vi "sever-client.vi"() -> ()   [LabVIEW 2020]
uses:
  <vilib>/Utility/sysdir.llb/System Directory Type.ctl
panel:
  in  "s 6":bool=TRUE
  in  "s 5":bool
  in  "s 4":bool=TRUE
  in  "批量发送菜单":bool
  out "接收数据":string
  in  "发送数据":string
  out "远程端口":u16
  out "远程地址":string
  in  "批量发送":string[][](table)=[["Date", "Delay(ms)"], ["", ""], ["", ""], ["", ""], ["", ""], ["", ""]]
  in  "定时间隔毫秒":dbl
  in  "定时发送":bool
  out "当前发送":string
  out "数值":dbl
  out "times":dbl
  in  "s 3":bool
  out "添加的路径":path
  out "每小时读码次数":dbl
  in  "s 2":bool
  out "时间统计":string
  in  "s":bool
  out "total times":dbl
  out "standard output":string caption="PING标准输出"
  in  "停止":bool
  in  "开启检测模式":bool
  out "误码次数":dbl
  in  "标准码词":string="\r"
  in  "十六进制显示":bool=TRUE
  in  "自动换行":bool=TRUE
  in  "时间显示":bool=TRUE
  in  "接收超时毫秒":i32=200
  in  "清空接收数据区":bool
  in  "读取的字节":i32=300
  in  "十六进制发送":bool=TRUE
  in  "清空发送数据区":bool
  in  "发送超时毫秒":i32=200
  in  "发送":bool
  in  "数据保存":bool
  in  "路径":path
  in  "服务器IP地址":string="192.168.1.103"
  in  "sever-client":u16(ring) items=["TCP-Sever", "TCP-client"]
  in  "服务器端口号":u16=34567
  in  "开始":bool
  out "错误输出":errorcluster caption="TCP错误输出"
  # "V1.0.1"
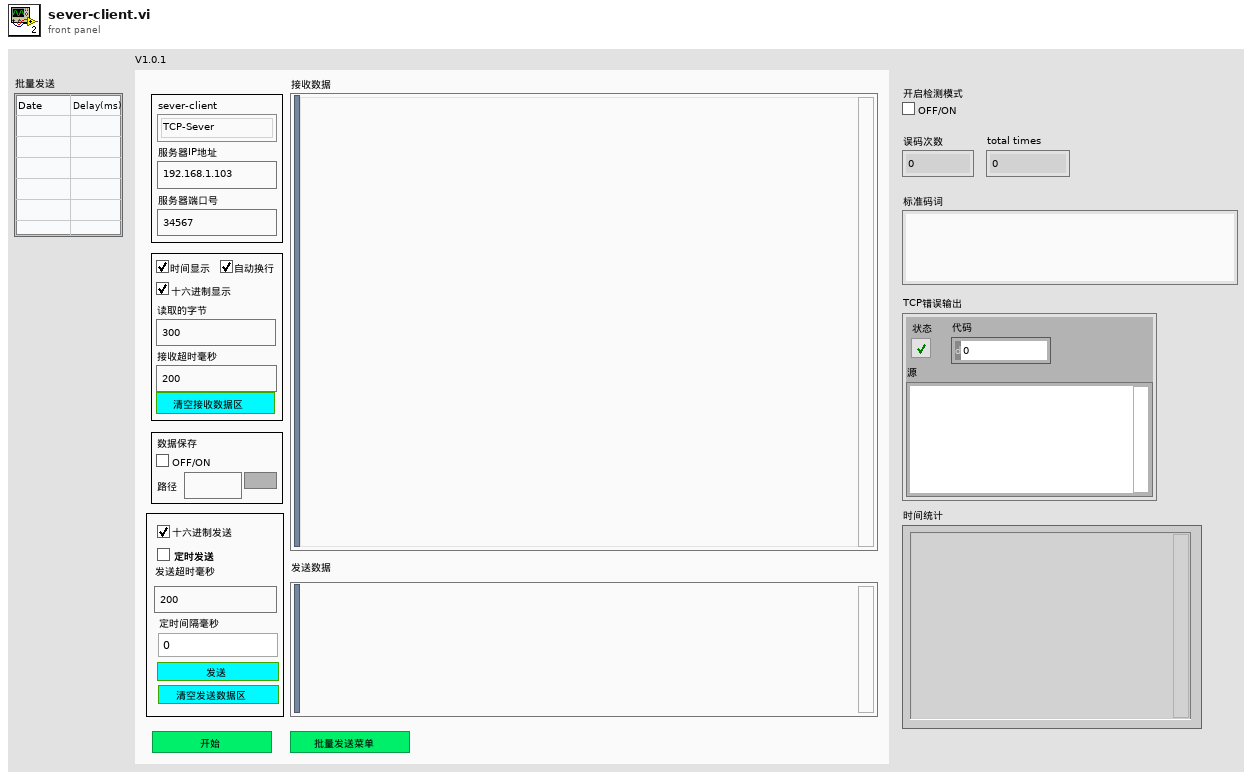
[diagram p1: front panel]
types:
  T1 = typedef "System Directory Type.ctl" = i32
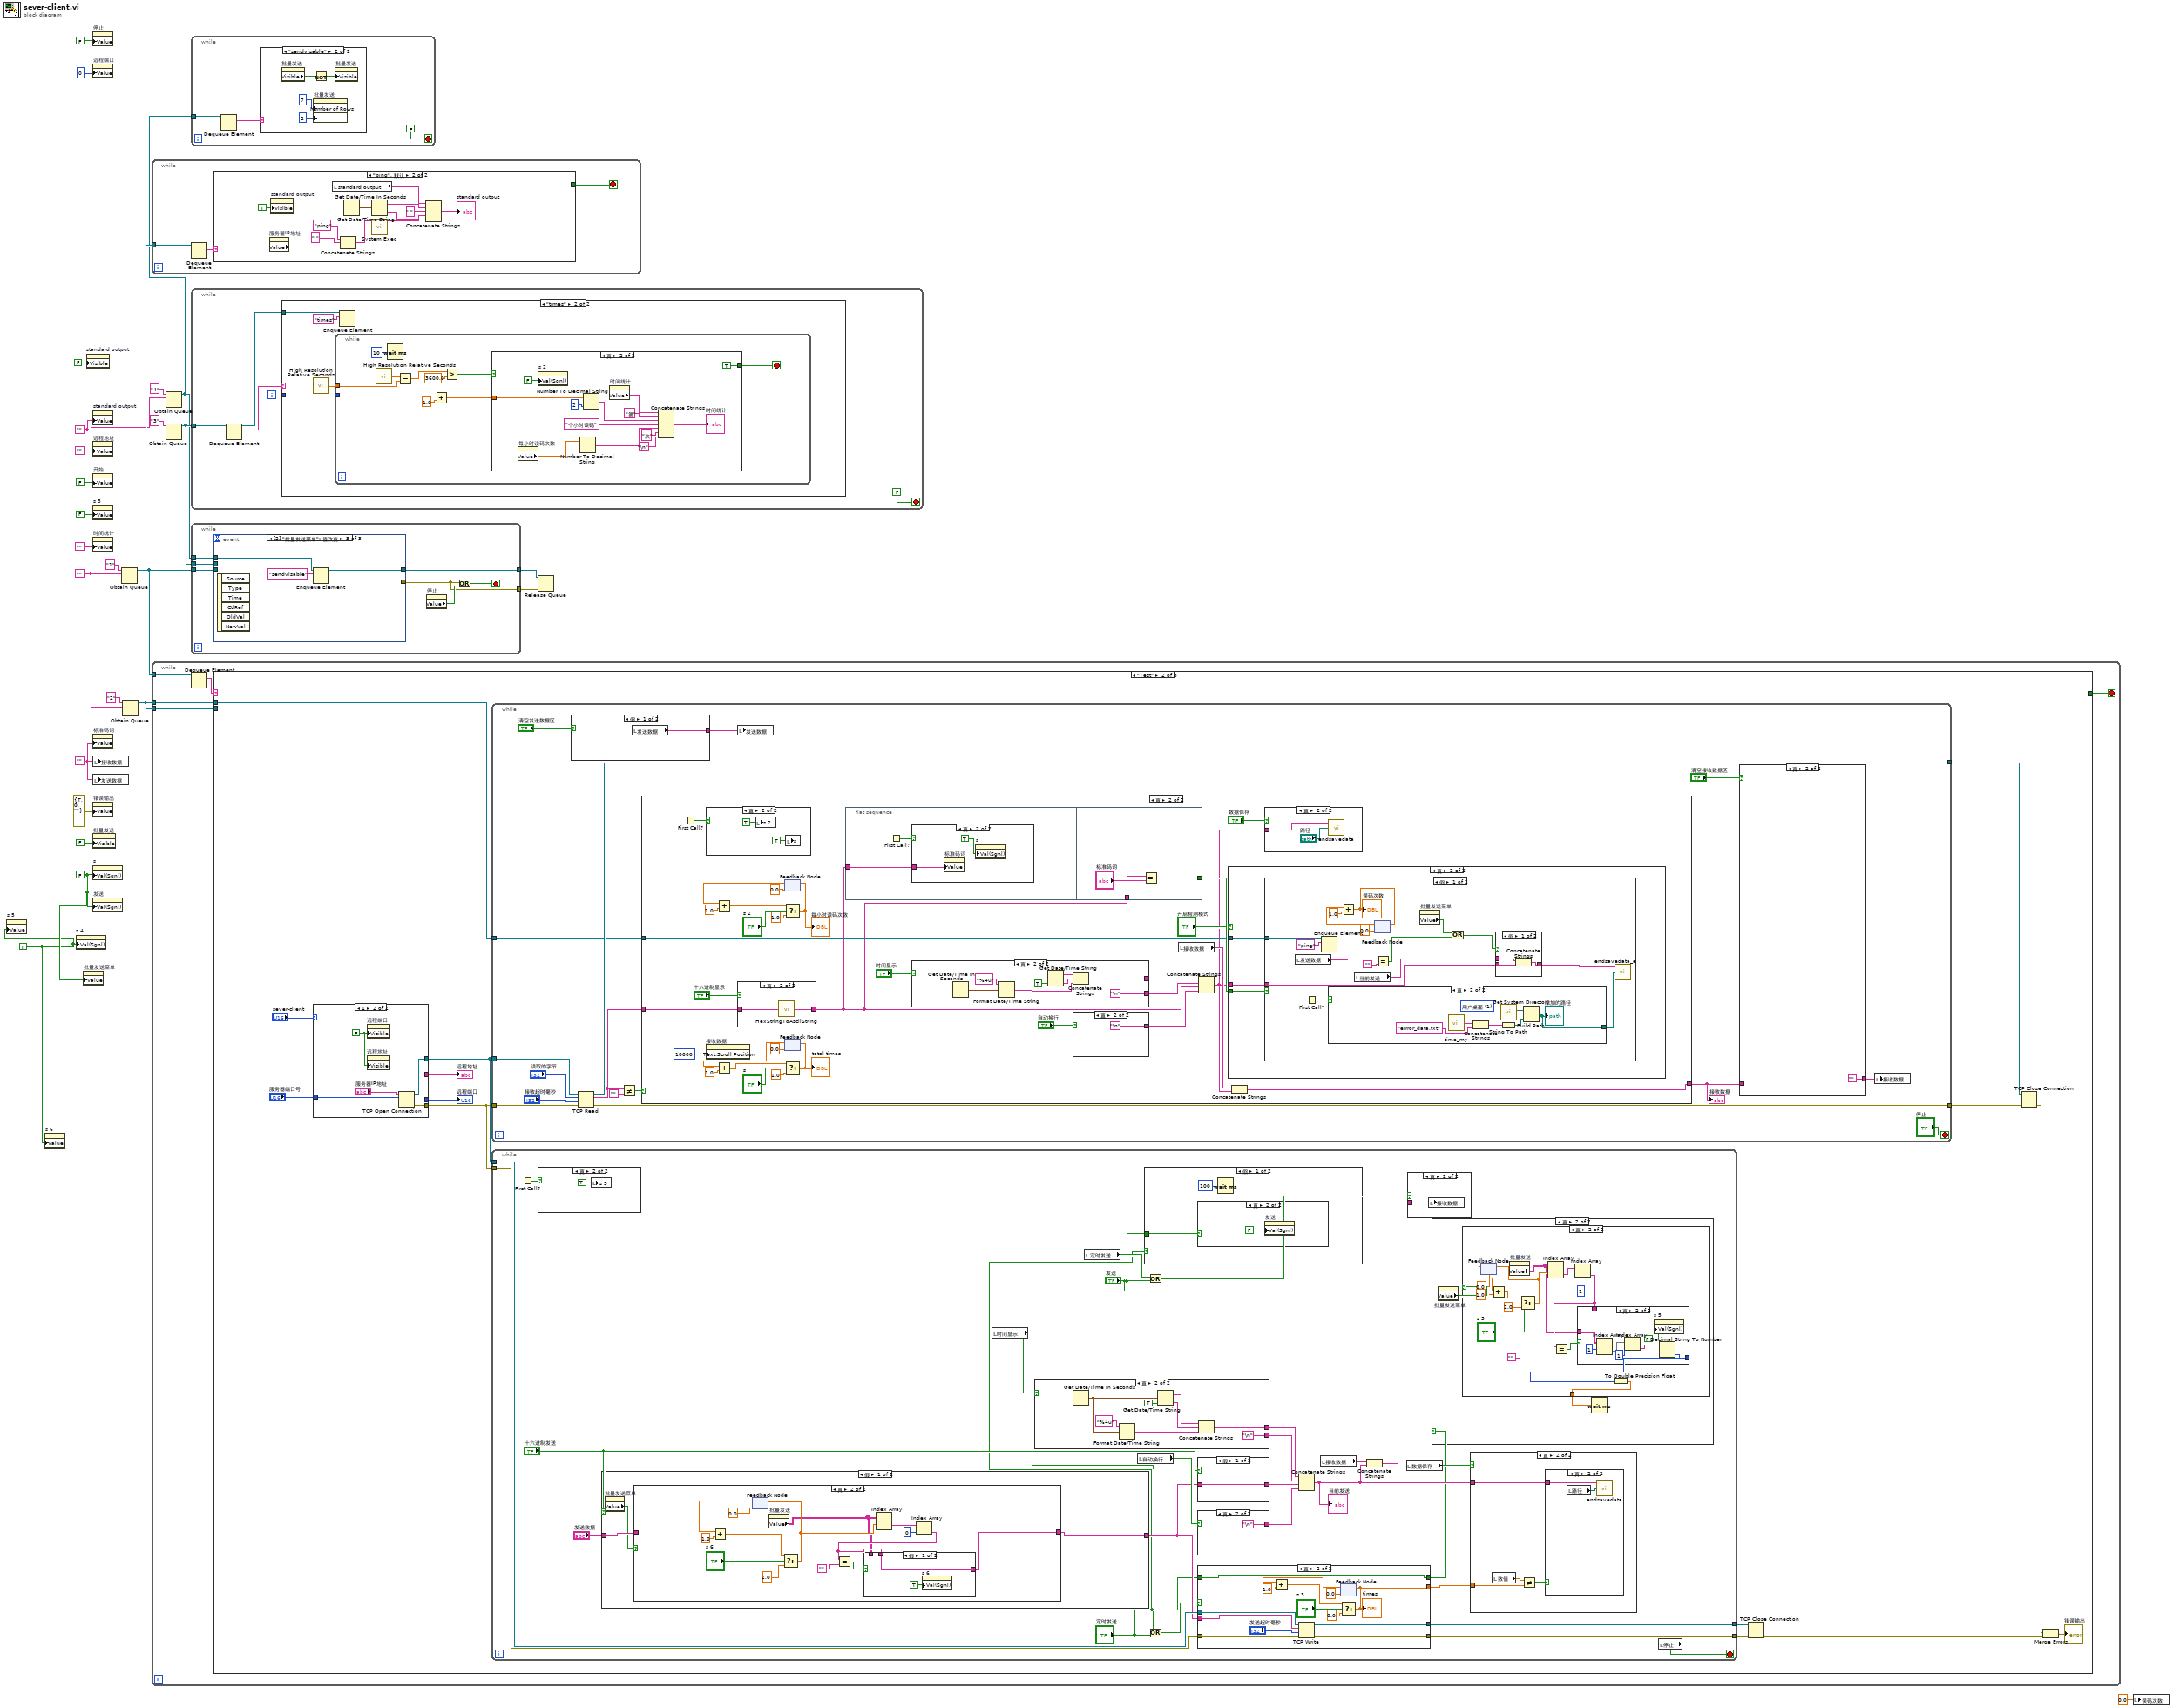
[diagram p0: block diagram]
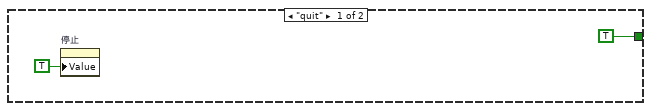
[diagram p5: hidden frame]
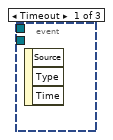
[diagram p6: hidden frame]
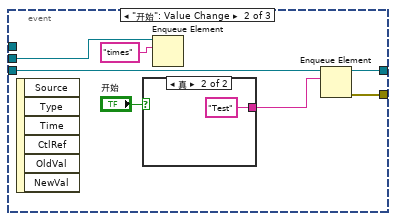
[diagram p7: hidden frame]
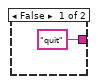
[diagram p8: hidden frame]
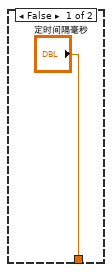
[diagram p13: hidden frame]
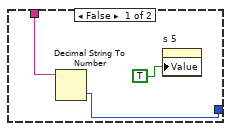
[diagram p14: hidden frame]
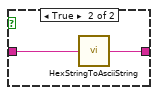
[diagram p17: hidden frame]
diagram:
  w1 = TRUE ("值(信号)")
  w8 = ""
  w3 = FALSE ("值(信号)")
  w12 = ""
  w5 = ""
  n1 = property on="s 5" class="Bool (严格)"("Value"=w1) -> ()  [unwired: 2 in, 2 out]
  n2 = property on="s 6" class="Bool (严格)"("Value"=w1) -> ()  [unwired: 2 in, 2 out]
  n3 = property on="s 4" class="Bool (严格)"("Val(Sgnl)"=w1) -> ()  [unwired: 2 in, 2 out]
  n4 = property on="批量发送菜单" class="Bool (严格)"("Value"=w3) -> ()  [unwired: 2 in, 2 out]
  n5 = property on="standard output" class="Str"("Visible"=FALSE ("可见")) -> ()  [unwired: 2 in, 2 out]
  n6 = property on="停止" class="Bool (严格)"("Value"=FALSE ("停止")) -> ()  [unwired: 2 in, 2 out]
  n7 = property on="远程端口" class="DigNum (严格)"("Value"=u16 0 ("远程端口")) -> ()  [unwired: 2 in, 2 out]
  n8 = property on="standard output" class="Str"("Value"=w12) -> ()  [unwired: 2 in, 2 out]
  n9 = property on="远程地址" class="Str"("Value"="") -> ()  [unwired: 2 in, 2 out]
  n10 = property on="开始" class="Bool (严格)"("Value"=FALSE ("开始")) -> ()  [unwired: 2 in, 2 out]
  n11 = property on="s 3" class="Bool (严格)"("Value"=FALSE ("s 3")) -> ()  [unwired: 2 in, 2 out]
  n12 = property on="时间统计" class="Str"("Value"="") -> ()  [unwired: 2 in, 2 out]
  n13 = property on="标准码词" class="Str"("Value"=w8) -> ()  [unwired: 2 in, 2 out]
  n14 = local write "接收数据"(w8) -> ()
  n15 = local write "发送数据"(w8) -> ()
  n16 = property on="错误输出" class="Clust (严格)"("Value"=errorcluster {"status"=TRUE, "code"=0, "source"=""} ("错误输出")) -> ()  [unwired: 2 in, 2 out]
  n17 = property on="批量发送" class="Tbl (严格)"("Visible"=FALSE ("可见")) -> ()  [unwired: 2 in, 2 out]
  n18 = property on="s" class="Bool (严格)"("Val(Sgnl)"=w3) -> ()  [unwired: 2 in, 2 out]
  n19 = property on="发送" class="Bool (严格)"("Val(Sgnl)"=w3) -> ()  [unwired: 2 in, 2 out]
  n20 = Obtain Queue(name (unnamed)="1" ("名称（未命名）"), element data type=w5) -> (queue out=w24:refnum<queue>)  [unwired: 3 in, 2 out]
  n21 = Obtain Queue(name (unnamed)="2" ("名称（未命名）"), element data type=w5) -> (queue out=w20:refnum<queue>)  [unwired: 3 in, 2 out]
  n22 = while {
    tunnel: w20 -> [w26]
    stop <- w27 stop-if-true
    n23 = Dequeue Element(queue=w26) -> (element=w28:string)  [unwired: 2 in, 3 out]
    n24 = case shown="\"ping\", 默认" w28 {
      tunnel: [TRUE _] -> w27
      frame "quit" {
        n25 = property on="停止" class="Bool (严格)"("Value"=TRUE ("停止")) -> ()  [unwired: 2 in, 2 out]
      }
      frame "ping", Default {
        n26 = property on="服务器IP地址" class="Str"() -> ("Value"=w40:string)  [unwired: 2 in, 2 out]
        n27 = property on="standard output" class="Str"("Visible"=TRUE ("可见")) -> ()  [unwired: 2 in, 2 out]
        n28 = local read "standard output"() -> (w32:string)
        n29 = Concatenate Strings("ping" ("字符串"), " " ("字符串"), w40) -> (w39:string)
        n30 = Get Date/Time In Seconds() -> (seconds since 1Jan1904=w37:timestamp)
        n31 = call <vilib>:"System Exec.vi"("command line"=w39) -> ("standard output"=w38:string)  [unwired: 7 in, 3 out]
        n32 = Get Date/Time String(seconds (now)=w37) -> (date string=w36:string, time string=w34:string)  [unwired: 2 in]
        n33 = Concatenate Strings(w32, w36, " " ("字符串"), w34, w38) -> (→"standard output":string)
      }
    }
  }
  n34 = while {
    tunnel: w24 -> [w45]
    tunnel: w20 -> [w44]
    tunnel: w20 -> [w43]
    stop <- w47 stop-if-true
    n35 = Dequeue Element(queue=w45) -> (element=w46:string)  [unwired: 2 in, 3 out]
    n36 = case shown="\"Test\"" w46 {
      tunnel: [_ _ TRUE] -> w47
      tunnel: w44 -> [_ w56 _]
      tunnel: w43 -> [_ _ w338]
      frame "假", Default {
      }
      frame "Test" {
        n37 = case shown="1" "sever-client" {
          tunnel: "服务器端口号" -> [w221 w226]
          tunnel: [w220 w225] -> w55
          tunnel: [w219 w224] -> w54
          tunnel: [w218 _] -> w59
          tunnel: [w217 _] -> w58
          frame 0, Default {
            w216 = TRUE
            n38 = property on="远程端口" class="DigNum (严格)"("Visible"=w216) -> ()  [unwired: 2 in, 2 out]
            n39 = property on="远程地址" class="Str"("Visible"=w216) -> ()  [unwired: 2 in, 2 out]
            n40 = call <vilib>:"TCP Listen.vi"("port"=w221) -> ("error out"=w219:errorcluster, "remote port"=w217:u16, "remote address"=w218:string, "connection ID"=w220:refnum<k5>)  [unwired: 6 in, 1 out]
          }
          frame 1 {
            w222 = FALSE
            n41 = property on="远程端口" class="DigNum (严格)"("Visible"=w222) -> ()  [unwired: 2 in, 2 out]
            n42 = property on="远程地址" class="Str"("Visible"=w222) -> ()  [unwired: 2 in, 2 out]
            n43 = TCP Open Connection(address="服务器IP地址", remote port or service name=w226) -> (connection ID=w225:refnum<k5>, error out=w224:errorcluster)  [unwired: 3 in]
          }
        }
        "远程地址" <- w59
        "远程端口" <- w58
        n44 = while {
          tunnel: [w240] -> w49
          tunnel: [w232] -> w57
          tunnel: w56 -> [w231]
          tunnel: w55 -> [w229]
          tunnel: w54 -> [w228]
          stop <- "停止" stop-if-true
          n45 = case shown="假" "清空发送数据区" {
            tunnel: [w243 ""] -> w233
            frame False {
              n46 = local read "发送数据"() -> (w243:string)
            }
            frame True {
            }
          }
          n47 = TCP Read(connection ID=w229, bytes to read="读取的字节", error in (no error)=w228, 9:"接收超时毫秒") -> (connection ID out=w240:refnum<k5>, data out=w238:string, error out=w232:errorcluster)  [unwired: 1 in]
          n48 = Not Equal?(x=w238, y="") -> (x != y?=w227:bool)
          n49 = case shown="真" w227 {
            tunnel: w238 -> [_ w278]
            tunnel: [w252 w280] -> w235
            tunnel: w231 -> [_ w274]
            frame False {
              n50 = local read "接收数据"() -> (w252:string)
            }
            frame True {
              n51 = First Call?() -> (First Call?: T/F=w253:bool)
              n52 = case shown="真" w253 {
                frame False {
                }
                frame True {
                  n53 = local write "s 2"(TRUE ("值(信号)")) -> ()
                  n54 = local write "s"(TRUE ("值(信号)")) -> ()
                }
              }
              n55 = property on="接收数据" class="Str"("Text.Scroll Position"=u32 10000 ("文本.滚动条位置")) -> ()  [unwired: 2 in, 2 out]
              n56 = case shown="真" "十六进制显示" {
                tunnel: [w324 w326] -> w256
                tunnel: w278 -> [w324 w325]
                frame False {
                }
                frame True {
                  n57 = call "HexStringToAsciiString.vi"("输入Hex字符串"=w325) -> ("输出Ascii"=w326:string)
                }
              }
              n58 = feedback #1(0.0 ("x")) -> (w263:dbl)
              n59 = Add(x=w263, y=1.0) -> (x+y=w264:dbl)
              n60 = Select(t=w264, s="s 2", f=1.0) -> (s? t:f=w259:dbl)
              "每小时读码次数" <- w259
              n61 = feedback-in #1(w259) -> ()
              n62 = feedback #2(0.0 ("x")) -> (w270:dbl)
              n63 = Add(x=w270, y=1.0) -> (x+y=w269:dbl)
              n64 = Select(t=w269, s="s", f=1.0) -> (s? t:f=w266:dbl)
              "total times" <- w266
              n65 = feedback-in #2(w266) -> ()
              n66 = flat-sequence {
                tunnel: w256 -> [w286]
                tunnel: w256 -> [w290]
                tunnel: [w291] -> w277
                frame #0 {
                  n67 = First Call?() -> (First Call?: T/F=w287:bool)
                  n68 = case shown="真" w287 {
                    tunnel: w286 -> [_ w289]
                    frame False {
                    }
                    frame True {
                      n69 = property on="标准码词" class="Str"("Value"=w289) -> ()  [unwired: 2 in, 2 out]
                      n70 = property on="s" class="Bool (严格)"("Val(Sgnl)"=TRUE ("值(信号)")) -> ()  [unwired: 2 in, 2 out]
                    }
                  }
                }
                frame #1 {
                  n71 = Equal?(x=w290, y="标准码词") -> (x = y?=w291:bool)
                }
              }
              n72 = case shown="真" "时间显示" {
                tunnel: [_ w334] -> w258
                tunnel: [_ "\n"] -> w257
                frame False {
                }
                frame True {
                  n73 = Get Date/Time In Seconds() -> (seconds since 1Jan1904=w331:timestamp)
                  n74 = Format Date/Time String(time format string (%c)="%4u" ("时间格式字符串(%c)"), seconds (now)=w331) -> (date/time string=w330:string)  [unwired: 1 in]
                  n75 = Get Date/Time String(want seconds? (F)=TRUE ("需要秒？(F)")) -> (date string=w336:string, time string=w335:string)  [unwired: 2 in]
                  n76 = Concatenate Strings(w336, w335, w330) -> (w334:string)
                }
              }
              n77 = case shown="真" "自动换行" {
                tunnel: [_ "\n"] -> w255
                frame False {
                }
                frame True {
                }
              }
              n78 = local read "接收数据"() -> (w282:string)
              n79 = Concatenate Strings(w258, w257, w256, w255) -> (w254:string)
              n80 = case shown="真" "开启检测模式" {
                tunnel: w277 -> [_ w295]
                tunnel: w274 -> [_ w294]
                tunnel: w254 -> [_ w293]
                frame False {
                }
                frame True {
                  n81 = case shown="假" w295 {
                    tunnel: w294 -> [w306 _]
                    tunnel: w293 -> [w301 _]
                    frame False {
                      n82 = local read "发送数据"() -> (w299:string)
                      n83 = First Call?() -> (First Call?: T/F=w305:bool)
                      n84 = Enqueue Element(queue=w306, element="ping" ("元素")) -> ()  [unwired: 2 in, 3 out]
                      n85 = case shown="真" w305 {
                        tunnel: [w316 w319] -> w304
                        frame False {
                          n86 = local read "添加的路径"() -> (w316:path)
                        }
                        frame True {
                          w323 = T1 1 items=["用户目录"=0, "用户桌面"=1, "用户文档"=2, "用户应用程序数据"=3, "用户设置"=4, "用户临时目录"=5, "公共文档"=6, "公共应用程序数据"=7, "公共设置"=8, "公共缓存"=13, "系统核心库"=9, "系统安装库"=10, "应用程序文件"=11, "启动盘根目录"=12] ("system directory type")
                          n87 = call "time_my.vi"() -> ("时间"=w317:string)
                          n88 = Concatenate Strings(w317, "errror_data.txt") -> (w321:string)
                          n89 = call <vilib>:"Get System Directory.vi"("system directory type"=w323) -> ("system directory"=w322:path)  [unwired: 10 in]
                          n90 = String To Path(string=w321) -> (path=w320:path)
                          n91 = Build Path(base path=w322, name or relative path=w320) -> (appended path=w319:path)
                          "添加的路径" <- w319
                        }
                      }
                      n92 = local read "当前发送"() -> (w300:string)
                      n93 = feedback #3(0.0) -> (w308:dbl)
                      n94 = Add(x=w308, y=1.0) -> (x+y=w310:dbl)
                      "误码次数" <- w310
                      n95 = feedback-in #3(w310) -> ()
                      n96 = Equal?(x=w299, y="") -> (x = y?=w298:bool)
                      n97 = property on="批量发送菜单" class="Bool (严格)"() -> ("Value"=w297:bool)  [unwired: 2 in, 2 out]
                      n98 = Or(x=w297, y=w298) -> (x .or. y?=w296:bool)
                      n99 = case shown="假" w296 {
                        tunnel: [w314 w315] -> w302
                        tunnel: w301 -> [w313 w315]
                        tunnel: w300 -> [w312 _]
                        frame False {
                          n100 = Concatenate Strings(w312, w313) -> (w314:string)
                        }
                        frame True {
                        }
                      }
                      n101 = call "endsavedata_e.vi"("文件路径（使用对话框）"=w304, "文本"=w302) -> ()  [unwired: 1 in, 2 out]
                    }
                    frame True {
                    }
                  }
                }
              }
              n102 = Concatenate Strings(w282, w254) -> (w280:string)
              n103 = case shown="真" "数据保存" {
                tunnel: w254 -> [_ w327]
                frame False {
                }
                frame True {
                  n104 = call "endsavedata.vi"("文件路径（使用对话框）"="路径", "文本"=w327) -> ()  [unwired: 1 in, 2 out]
                }
              }
            }
          }
          "接收数据" <- w235
          n105 = local write "发送数据"(w233) -> ()
          n106 = case shown="真" "清空接收数据区" {
            tunnel: [w248 ""] -> w237
            tunnel: w235 -> [w246 _]
            frame False {
              n107 = String Length(string=w246) -> (length=w250:i32)
              n108 = Greater?(x=w250, y=10000) -> (0:w249:bool)
              n109 = Select(t="", s=w249, f=w246) -> (s? t:f=w248:string)
            }
            frame True {
            }
          }
          n110 = local write "接收数据"(w237) -> ()
        }
        n111 = while {
          tunnel: w55 -> [w87]
          tunnel: w54 -> [w86]
          tunnel: [w85] -> w53
          tunnel: [w68] -> w48
          stop <- w84 stop-if-true
          n112 = First Call?() -> (First Call?: T/F=w72:bool)
          n113 = case shown="真" w72 {
            frame False {
            }
            frame True {
              n114 = local write "s 3"(TRUE ("s 3")) -> ()
            }
          }
          n115 = case shown="假" "十六进制发送" {
            selector: "十六进制发送" -> [_ w176]
            tunnel: "发送数据" -> [w152 w179]
            tunnel: [w151 w178] -> w77
            frame False {
              n116 = property on="批量发送菜单" class="Bool (严格)"() -> ("Value"=w150:bool)  [unwired: 2 in, 2 out]
              n117 = case shown="真" w150 {
                tunnel: [w153 w156] -> w151
                tunnel: w152 -> [w153 _]
                frame False {
                }
                frame True {
                  n118 = feedback #4(0.0 ("x")) -> (w164:dbl)
                  n119 = Add(x=w164, y=1.0) -> (x+y=w161:dbl)
                  n120 = property on="批量发送" class="Tbl (严格)"() -> ("Value"=w154:string[][])  [unwired: 2 in, 2 out]
                  n121 = Select(t=w161, s="s 6", f=2.0) -> (s? t:f=w160:dbl)
                  n122 = feedback-in #4(w160) -> ()
                  n123 = Index Array(array=w154, index (row)=w160) -> (element=w167:string[])  [unwired: 1 in]
                  n124 = Index Array(array=w167, index=0 ("索引")) -> (element=w155:string)
                  n125 = Equal?(x=w155, y="") -> (x = y?=w157:bool)
                  n126 = case shown="假" w157 {
                    tunnel: [w169 w173] -> w156
                    tunnel: w155 -> [w169 _]
                    tunnel: w154 -> [_ w175]
                    frame False {
                      n127 = property on="s 6" class="Bool (严格)"("Val(Sgnl)"=TRUE ("值(信号)")) -> ()  [unwired: 2 in, 2 out]
                    }
                    frame True {
                      n128 = Index Array(array=w175, index (row)=1 ("索引 (行)")) -> (element=w174:string[])  [unwired: 1 in]
                      n129 = Index Array(array=w174, index=0 ("索引")) -> (element=w173:string)
                      n130 = property on="s 6" class="Bool (严格)"("Val(Sgnl)"=FALSE ("值(信号)")) -> ()  [unwired: 2 in, 2 out]
                    }
                  }
                }
              }
            }
            frame True {
              n131 = local read "times"() -> (→"数值":dbl)
              n132 = case shown="真" "批量发送菜单" {
                tunnel: w179 -> [w182 _]
                tunnel: [w181 w193] -> w178
                tunnel: w176 -> [_ w192]
                frame False {
                  n133 = call "AsciiStringToHexString.vi"("输入Asciistring1"=w182) -> ("输出HexString"=w181:string)
                }
                frame True {
                  n134 = feedback #5(0.0 ("x")) -> (w195:dbl)
                  n135 = Add(x=w195, y=1.0) -> (x+y=w190:dbl)
                  n136 = Select(t=w190, s="s 4", f=2.0) -> (s? t:f=w189:dbl)
                  n137 = feedback-in #5(w189) -> ()
                  n138 = Index Array(array="批量发送", index (row)=w189) -> (element=w198:string[])  [unwired: 1 in]
                  n139 = Index Array(array=w198, index=0 ("索引")) -> (element=w184:string)
                  n140 = Equal?(x=w184, y="") -> (x = y?=w186:bool)
                  n141 = case shown="假" w186 {
                    tunnel: [w200 w204] -> w185
                    tunnel: w184 -> [w200 _]
                    tunnel: "批量发送" -> [_ w206]
                    frame False {
                      n142 = property on="s 4" class="Bool (严格)"("Val(Sgnl)"=TRUE ("值(信号)")) -> ()  [unwired: 2 in, 2 out]
                    }
                    frame True {
                      n143 = Index Array(array=w206, index (row)=1 ("索引 (行)")) -> (element=w205:string[])  [unwired: 1 in]
                      n144 = Index Array(array=w205, index=0 ("索引")) -> (element=w204:string)
                      n145 = property on="s 4" class="Bool (严格)"("Val(Sgnl)"=FALSE ("值(信号)")) -> ()  [unwired: 2 in, 2 out]
                    }
                  }
                  n146 = case shown="真" w192 {
                    tunnel: [w207 w209] -> w193
                    tunnel: w185 -> [w207 w208]
                    frame False {
                    }
                    frame True {
                      n147 = call "AsciiStringToHexString.vi"("输入Asciistring1"=w208) -> ("输出HexString"=w209:string)
                    }
                  }
                }
              }
            }
          }
          n148 = local read "时间显示"() -> (w69:bool)
          n149 = case shown="真" w69 {
            tunnel: [_ w130] -> w81
            tunnel: [_ "\n"] -> w80
            frame False {
            }
            frame True {
              n150 = Get Date/Time In Seconds() -> (seconds since 1Jan1904=w126:timestamp)
              n151 = Format Date/Time String(time format string (%c)="%4u" ("时间格式字符串(%c)"), seconds (now)=w126) -> (date/time string=w127:string)  [unwired: 1 in]
              n152 = Get Date/Time String(seconds (now)=w126, want seconds? (F)=TRUE ("需要秒？(F)")) -> (date string=w131:string, time string=w128:string)  [unwired: 1 in]
              n153 = Concatenate Strings(w131, w128, w127) -> (w130:string)
            }
          }
          n154 = local read "定时发送"() -> (w67:bool)
          n155 = local read "自动换行"() -> (w82:bool)
          n156 = case shown="假" "定时发送" {
            tunnel: "发送" -> [w89 _]
            frame False {
              n157 = case shown="真" w89 {
                frame False {
                }
                frame True {
                  n158 = property on="发送" class="Bool (严格)"("Val(Sgnl)"=FALSE ("值(信号)")) -> ()  [unwired: 2 in, 2 out]
                }
              }
              n159 = Wait (ms)(milliseconds to wait=u32 100 ("等待时间（毫秒）")) -> ()  [unwired: 1 out]
            }
            frame True {
            }
          }
          n160 = Or(x=w67, y="发送") -> (x .or. y?=w66:bool)
          n161 = Or(x="发送", y="定时发送") -> (x .or. y?=w65:bool)
          n162 = case shown="假" "十六进制发送" {
            tunnel: [w121 w123] -> w76
            tunnel: w77 -> [w121 w122]
            frame False {
            }
            frame True {
              n163 = call "HexStringToAsciiString.vi"("输入Hex字符串"=w122) -> ("输出Ascii"=w123:string)
            }
          }
          n164 = case shown="真" w82 {
            tunnel: [_ "\n"] -> w78
            frame False {
            }
            frame True {
            }
          }
          n165 = case shown="真" w65 {
            tunnel: w77 -> [_ w145]
            tunnel: [w135 w149] -> w68
            tunnel: [w134 w148] -> w85
            tunnel: w87 -> [w135 w147]
            tunnel: w86 -> [w134 w146]
            tunnel: [_ w138] -> w71
            tunnel: "定时发送" -> [w133 w137]
            tunnel: [w133 w137] -> w64
            frame False {
            }
            frame True {
              n166 = TCP Write(connection ID=w147, data in=w145, error in (no error)=w146, 9:"发送超时毫秒") -> (connection ID out=w149:refnum<k5>, error out=w148:errorcluster)  [unwired: 1 out]
              n167 = feedback #6(0.0 ("x")) -> (w139:dbl)
              n168 = Add(x=w139, y=1.0) -> (x+y=w144:dbl)
              n169 = Select(t=w144, s="s 3", f=0.0) -> (s? t:f=w138:dbl)
              "times" <- w138
              n170 = feedback-in #6(w138) -> ()
            }
          }
          n171 = Concatenate Strings(w81, w80, w76, w78) -> (w74:string)
          "当前发送" <- w74
          n172 = local read "接收数据"() -> (w79:string)
          n173 = Concatenate Strings(w79, w74) -> (w73:string)
          n174 = local read "数据保存"() -> (w70:bool)
          n175 = case shown="真" w66 {
            tunnel: w73 -> [_ w120]
            frame False {
            }
            frame True {
              n176 = local write "接收数据"(w120) -> ()
            }
          }
          n177 = case shown="真" w64 {
            frame False {
            }
            frame True {
              n178 = property on="批量发送菜单" class="Bool (严格)"() -> ("Value"=w91:bool)  [unwired: 2 in, 2 out]
              n179 = case shown="真" w91 {
                tunnel: ["定时间隔毫秒" w94] -> w92
                frame False {
                }
                frame True {
                  n180 = feedback #7(0.0 ("x")) -> (w104:dbl)
                  n181 = Add(x=w104, y=1.0) -> (x+y=w103:dbl)
                  n182 = property on="批量发送" class="Tbl (严格)"() -> ("Value"=w98:string[][])  [unwired: 2 in, 2 out]
                  n183 = Select(t=w103, s="s 5", f=2.0) -> (s? t:f=w99:dbl)
                  n184 = feedback-in #7(w99) -> ()
                  n185 = Index Array(array=w98, index (row)=w99) -> (element=w108:string[])  [unwired: 1 in]
                  n186 = Index Array(array=w108, index=1 ("索引")) -> (element=w102:string)
                  n187 = Equal?(x=w102, y="") -> (x = y?=w100:bool)
                  n188 = case shown="真" w100 {
                    tunnel: w102 -> [w111 _]
                    tunnel: [w110 w113] -> w95
                    tunnel: w98 -> [_ w117]
                    frame False {
                      n189 = Decimal String To Number(string=w111) -> (number=w110:i32)  [unwired: 2 in, 1 out]
                      n190 = property on="s 5" class="Bool (严格)"("Value"=TRUE ("s 5")) -> ()  [unwired: 2 in, 2 out]
                    }
                    frame True {
                      n191 = Index Array(array=w117, index (row)=1 ("索引 (行)")) -> (element=w116:string[])  [unwired: 1 in]
                      n192 = Index Array(array=w116, index=1 ("索引")) -> (element=w114:string)
                      n193 = property on="s 5" class="Bool (严格)"("Val(Sgnl)"=FALSE ("值(信号)")) -> ()  [unwired: 2 in, 2 out]
                      n194 = Decimal String To Number(string=w114) -> (number=w113:i32)  [unwired: 2 in, 1 out]
                    }
                  }
                  n195 = To Double Precision Float(number=w95) -> (double precision float=w94:dbl)
                }
              }
              n196 = Wait (ms)(milliseconds to wait=w92) -> ()  [unwired: 1 out]
            }
          }
          n197 = case shown="真" w70 {
            tunnel: w74 -> [_ w213]
            tunnel: w71 -> [_ w211]
            frame False {
            }
            frame True {
              n198 = local read "数值"() -> (w210:dbl)
              n199 = Not Equal?(x=w210, y=w211) -> (x != y?=w212:bool)
              n200 = case shown="真" w212 {
                tunnel: w213 -> [_ w214]
                frame False {
                }
                frame True {
                  n201 = local read "路径"() -> (w215:path)
                  n202 = call "endsavedata.vi"("文件路径（使用对话框）"=w215, "文本"=w214) -> ()  [unwired: 1 in, 2 out]
                }
              }
            }
          }
          n203 = local read "停止"() -> (w84:bool)
        }
        n204 = TCP Close Connection(connection ID=w48, error in (no error)=w53) -> (error out=w52:errorcluster)  [unwired: 1 in, 1 out]
        n205 = TCP Close Connection(connection ID=w49, error in (no error)=w57) -> (error out=w51:errorcluster)  [unwired: 1 in, 1 out]
        n206 = Merge Errors(w51, w52) -> (→"错误输出":errorcluster)
      }
      frame "quit" {
        n207 = Enqueue Element(queue=w338, element="quit" ("元素")) -> ()  [unwired: 2 in, 3 out]
      }
    }
  }
  n208 = Obtain Queue(name (unnamed)="4" ("名称（未命名）"), element data type=w5) -> (queue out=w6:refnum<queue>)  [unwired: 3 in, 2 out]
  n209 = Obtain Queue(name (unnamed)="3" ("名称（未命名）"), element data type=w12) -> (queue out=w14:refnum<queue>)  [unwired: 3 in, 2 out]
  n210 = while {
    tunnel: w6 -> [w342]
    stop <- FALSE stop-if-true
    n211 = Dequeue Element(queue=w342) -> (element=w343:string)  [unwired: 2 in, 3 out]
    n212 = case shown="\"sendvisable\"" w343 {
      frame "假", Default {
      }
      frame "sendvisable" {
        n213 = property on="批量发送" class="Tbl (严格)"() -> ("Visible"=w347:bool)  [unwired: 2 in, 2 out]
        n214 = Not(x=w347) -> (.not. x?=w346:bool)
        n215 = property on="批量发送" class="Tbl (严格)"("Number of Rows"=u32 7 ("行数"), "Number of Columns"=u32 2 ("列数")) -> ()  [unwired: 2 in, 2 out]
        n216 = property on="批量发送" class="Tbl (严格)"("Visible"=w346) -> ()  [unwired: 2 in, 2 out]
      }
    }
  }
  n217 = while {
    tunnel: w14 -> [w350]
    i -> [w349]
    stop <- FALSE stop-if-true
    n218 = Dequeue Element(queue=w350) -> (queue out=w348:refnum<queue>, element=w351:string)  [unwired: 2 in, 2 out]
    n219 = case shown="\"times\"" w351 {
      tunnel: w349 -> [_ w355]
      tunnel: w348 -> [_ w354]
      frame "假", Default {
      }
      frame "times" {
        n220 = call <vilib>:"High Resolution Relative Seconds.vi"() -> ("relative seconds"=w356:dbl)
        n221 = while {
          tunnel: w356 -> [w365]
          tunnel: w355 -> [w358]
          stop <- w361 stop-if-true
          n222 = call <vilib>:"High Resolution Relative Seconds.vi"() -> ("relative seconds"=w366:dbl)
          n223 = Wait (ms)(milliseconds to wait=u32 10 ("等待时间（毫秒）")) -> ()  [unwired: 1 out]
          n224 = Subtract(x=w366, y=w365) -> (x-y=w364:dbl)
          n225 = Add(x=w358, y=1.0) -> (x+y=w357:dbl)
          n226 = Greater?(x=w364, y=3600.0) -> (0:w362:bool)
          n227 = case shown="真" w362 {
            tunnel: [_ TRUE] -> w361
            tunnel: w357 -> [_ w374]
            frame False {
            }
            frame True {
              n228 = property on="每小时读码次数" class="DigNum (严格)"() -> ("Value"=w371:dbl)  [unwired: 2 in, 2 out]
              n229 = property on="s 2" class="Bool (严格)"("Val(Sgnl)"=FALSE ("s 2")) -> ()  [unwired: 2 in, 2 out]
              n230 = Number To Decimal String(number=w371) -> (decimal integer string=w370:string)  [unwired: 1 in]
              n231 = Number To Decimal String(number=w374, width (-)=i16 2 ("宽度(-)")) -> (decimal integer string=w373:string)
              n232 = property on="时间统计" class="Str"() -> ("Value"=w369:string)  [unwired: 2 in, 2 out]
              n233 = Concatenate Strings(w369, "第" ("字符串"), w373, "个小时读码" ("字符串"), w370, "次" ("字符串"), "\n") -> (→"时间统计":string)
            }
          }
        }
        n234 = Enqueue Element(queue=w354, element="times" ("元素")) -> ()  [unwired: 2 in, 3 out]
      }
    }
  }
  n235 = while {
    tunnel: w24 -> [w386]
    tunnel: [w383] -> w23
    tunnel: [w382] -> w22
    tunnel: w14 -> [w381]
    tunnel: w6 -> [w380]
    stop <- w384 stop-if-true
    n236 = event shown="[2] \"批量发送菜单\": 值改变" {
      selector: _ -> [_ _ _]
      dyn-events: _ -> [_ _ _]
      timeout: _ -> [_ _ _]
      tunnel: w386 -> [_ w393 _]
      tunnel: [_ w390 _] -> w382
      tunnel: [_ w389 w396] -> w383
      tunnel: w381 -> [_ w388 _]
      tunnel: w380 -> [_ _ w398]
      event Timeout {
        n237 = event-data() -> ()  [unwired: 1 in, 3 out]
      }
      event "开始": Value Change {
        n238 = event-data() -> ()  [unwired: 1 in, 6 out]
        n239 = case shown="真" "开始" {
          tunnel: ["quit" ("元素") "Test" ("元素")] -> w391
          frame False {
          }
          frame True {
          }
        }
        n240 = Enqueue Element(queue=w388, element="times" ("元素")) -> ()  [unwired: 2 in, 3 out]
        n241 = Enqueue Element(queue=w393, element=w391) -> (queue out=w389:refnum<queue>, error out=w390:errorcluster)  [unwired: 2 in, 1 out]
      }
      event "批量发送菜单": Value Change {
        n242 = event-data() -> ()  [unwired: 1 in, 6 out]
        n243 = Enqueue Element(queue=w398, element="sendvisable" ("元素")) -> (queue out=w396:refnum<queue>)  [unwired: 2 in, 2 out]
      }
    }
    n244 = property on="停止" class="Bool (严格)"() -> ("Value"=w385:bool)  [unwired: 2 in, 2 out]
    n245 = Or(x=w382, y=w385) -> (x .or. y?=w384:bool)
  }
  n246 = Release Queue(queue=w23, error in (no error)=w22) -> ()  [unwired: 1 in, 3 out]
  n247 = local write "误码次数"(0.0 ("误码次数")) -> ()
